vi "ni579x Configure Amplifier.vi"(0 "Register Bus":T1, 1 "scope":string(combo)="rx", 5 "enable?":bool=TRUE, 11 "Error In":errorcluster) -> (4 "Register Bus (out)":T1, 6 "coerced enable":bool, 15 "Error Out":errorcluster)   [LabVIEW 2015, in "ni579x Config v2 Host.lvlib"]
uses:
  <instrlib>/ni579x/Config/v2/Host/ni579x Config v2 Host.lvlib
  <instrlib>/_niInstr/Register Bus/v0/Host/Public/Register Bus Session.ctl
  <instrlib>/_niInstr/Register Bus/v0/Host/Private/Session Data.ctl
  <instrlib>/_niInstr/Register Bus/v0/Host/niInstr Register Bus v0 Host.lvlib
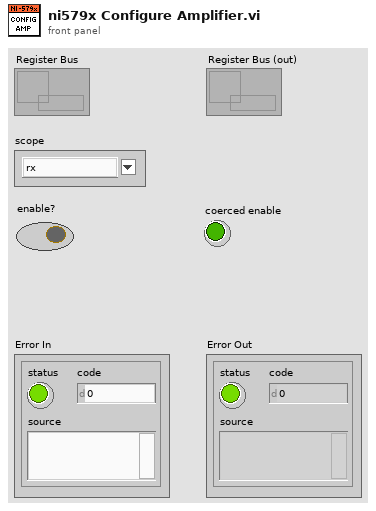
[diagram p1: front panel]
types:
  T1 = typedef "niInstr Register Bus v0 Host.lvlib/Register Bus Session.ctl" = refnum<queue>
  T2 = typedef "ni579x Config v2 Shared.lvlib/ni579x User Command.ctl" = cluster{"User Data 0":u8, "User Data 1":u8, "User Command ID":T3}
  T3 = typedef "ni579x Config v2 Shared.lvlib/ni579x User Command ID.ctl" = u8
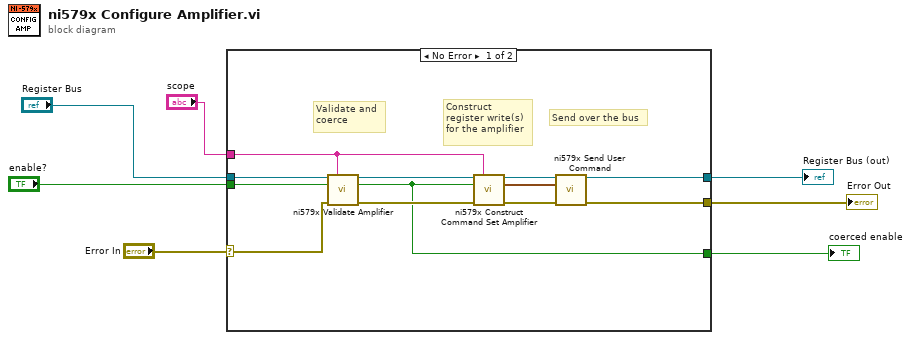
[diagram p0: block diagram]
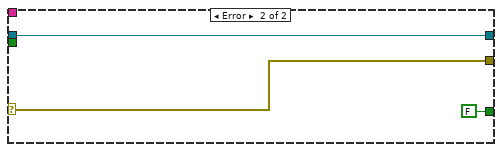
[diagram p2: hidden frame]
diagram:
  n1 = case shown="No Error" "Error In" {
    selector: "Error In" -> [w18 w22]
    tunnel: [w16 w22] -> w6
    tunnel: "Register Bus" -> [w19 w21]
    tunnel: "enable?" -> [w9 _]
    tunnel: [w17 w21] -> w4
    tunnel: "scope" -> [w12 _]
    tunnel: [w8 FALSE ("coerced enable")] -> w1
    frame No Error {
      # "Construct\nregister write(s)\nfor the amplifier"
      # "Send over the bus"
      # "Validate and \ncoerce"
      n2 = call <instrlib>:"ni579x Validate Amplifier.vi"("Register Bus"=w19, "scope"=w12, "enable?"=w9, "Error In"=w18) -> ("Register Bus (out)"=w11:T1, "coerced enable"=w8:bool, "Error Out"=w10:errorcluster)  [unwired: 9 in]
      n3 = call <instrlib>:"ni579x Construct Command Set Amplifier.vi"("Register Bus"=w11, "scope"=w12, "enabled?"=w8, "Error In"=w10) -> ("Register Bus (out)"=w15:T1, "User Command"=w14:T2, "Error Out"=w13:errorcluster)  [unwired: 9 in]
      n4 = call <instrlib>:"ni579x Send User Command.vi"("Register Bus"=w15, "User Command"=w14, "Error In"=w13) -> ("Register Bus (out)"=w17:T1, "Error Out"=w16:errorcluster)  [unwired: 8 in, 3 out]
    }
    frame Error {
    }
  }
  "Register Bus (out)" <- w4
  "Error Out" <- w6
  "coerced enable" <- w1
